vi "Data_get.vi"() -> ()   [LabVIEW 2009]
uses:
  <vilib>/Analysis/2dsp.llb/Real FFT.vi
  <vilib>/Analysis/NI_AALPro.lvlib
panel:
  in  "FFT every#":u32=1 min=1 max=1000 step=1
  in  "#steps":u32
  in  "f step (MHz)":dbl=0.0003 min=0.00025 max=67.0 step=1e-06 format="%#.12f"
  in  "ps/point":T1(ring)
  in  "ns/div":T2(ring)
  out "Current sweep":u32=1 min=1 max=1000 step=1
  in  "Ext":string="ccd"
  out "f cur. (MHz)":string
  in  "Name":string="trace"
  in  "Folder":path
  in  "#Sweeps":u32=1 min=1 max=1000 step=1
  in  "Ampl. (dBm)":dbl min=-135.0 max=30.0 step=0.5 format="%#_8g"
  in  "f start (MHz)":dbl=0.0003 min=0.00025 max=67.0 step=1e-06 format="%#.12f"
  in  "Start":bool
  in  "Quit":bool
  in  "E8257D VISA Port":refnum<visa-resource-name>="GPIB0::1::INSTR"
  out "read time (ms)":u32
  out "#points":u32
  out "Busy":bool
  in  "Repetition rate (Hz)":ext=2.5
  in  "Chirp start (MHz)":ext=2.5
  in  "Filter up to (MHz)":ext=2.5
  in  "Amount of averagings":u32=10
  out "Data":dbl[](array[numeric])
  out "XY Graph 5":cluster{ext[], dbl[]}(graph)
  out "FFT (Im)":dbl[](array[numeric])
  out "FFT (Re)":dbl[](array[numeric])
  out "Final array":ext[][](array[numeric])
  out "size(s)":i32
  out "Oscilloscope Data":dbl[](array[numeric])
  in  "Channel Number":u16=1
  out "Oscilloscope graph":dbl[](graph)
  in  "Stop":bool
  in  "TDS VISA Port":refnum<visa-resource-name>="GPIB0::1::INSTR"
  # "TDS6000"
  # "E8257D"
  # "File Storage"
  # "Control"
  # "Spectrum data"
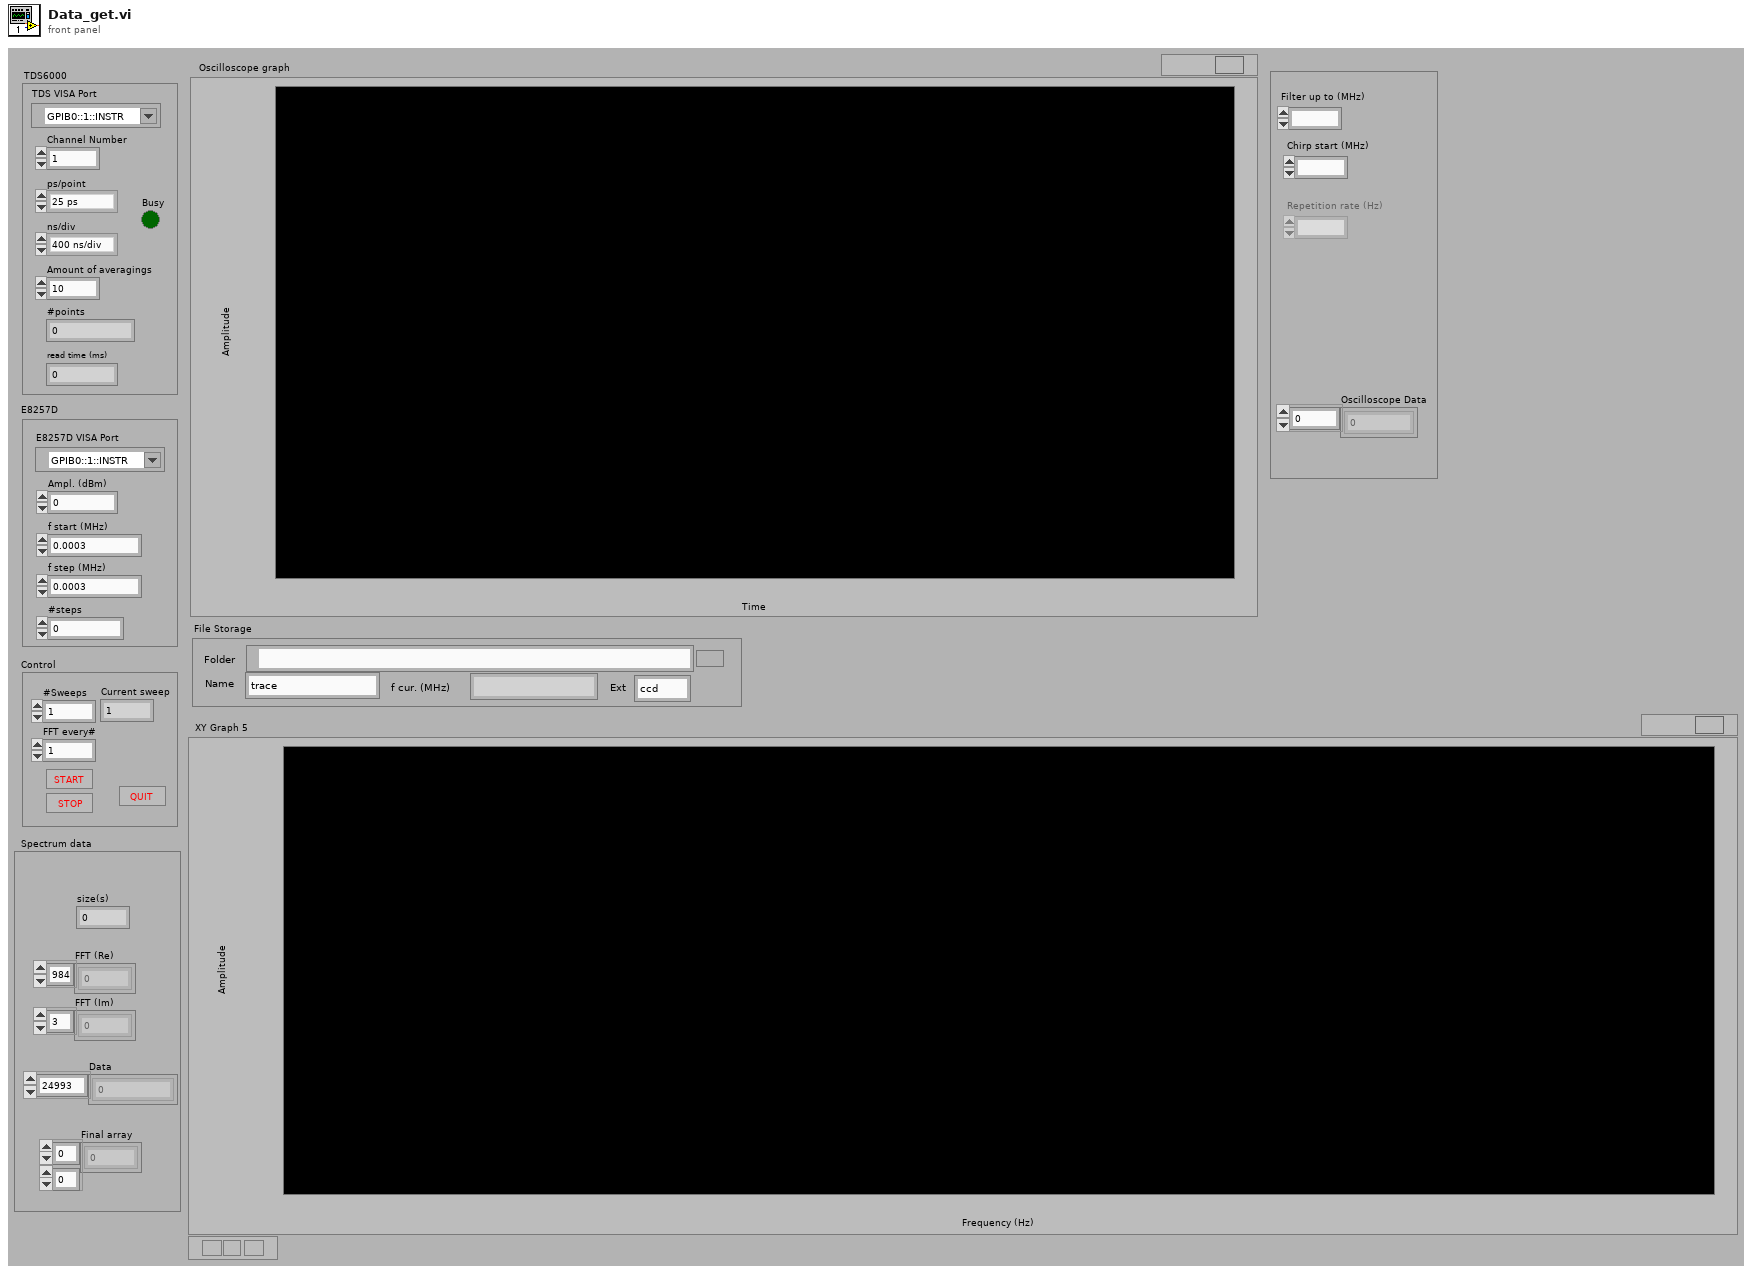
[diagram p1: front panel]
types:
  T1 = enum16{"25 ps", "50 ps", "100 ps", "200 ps", "400 ps", "800 ps", "2 ns"}
  T2 = enum16{"400 ns/div", "1 us/div", "2 us/div", "4 us/div", "10 us/div", "20 us/div"}
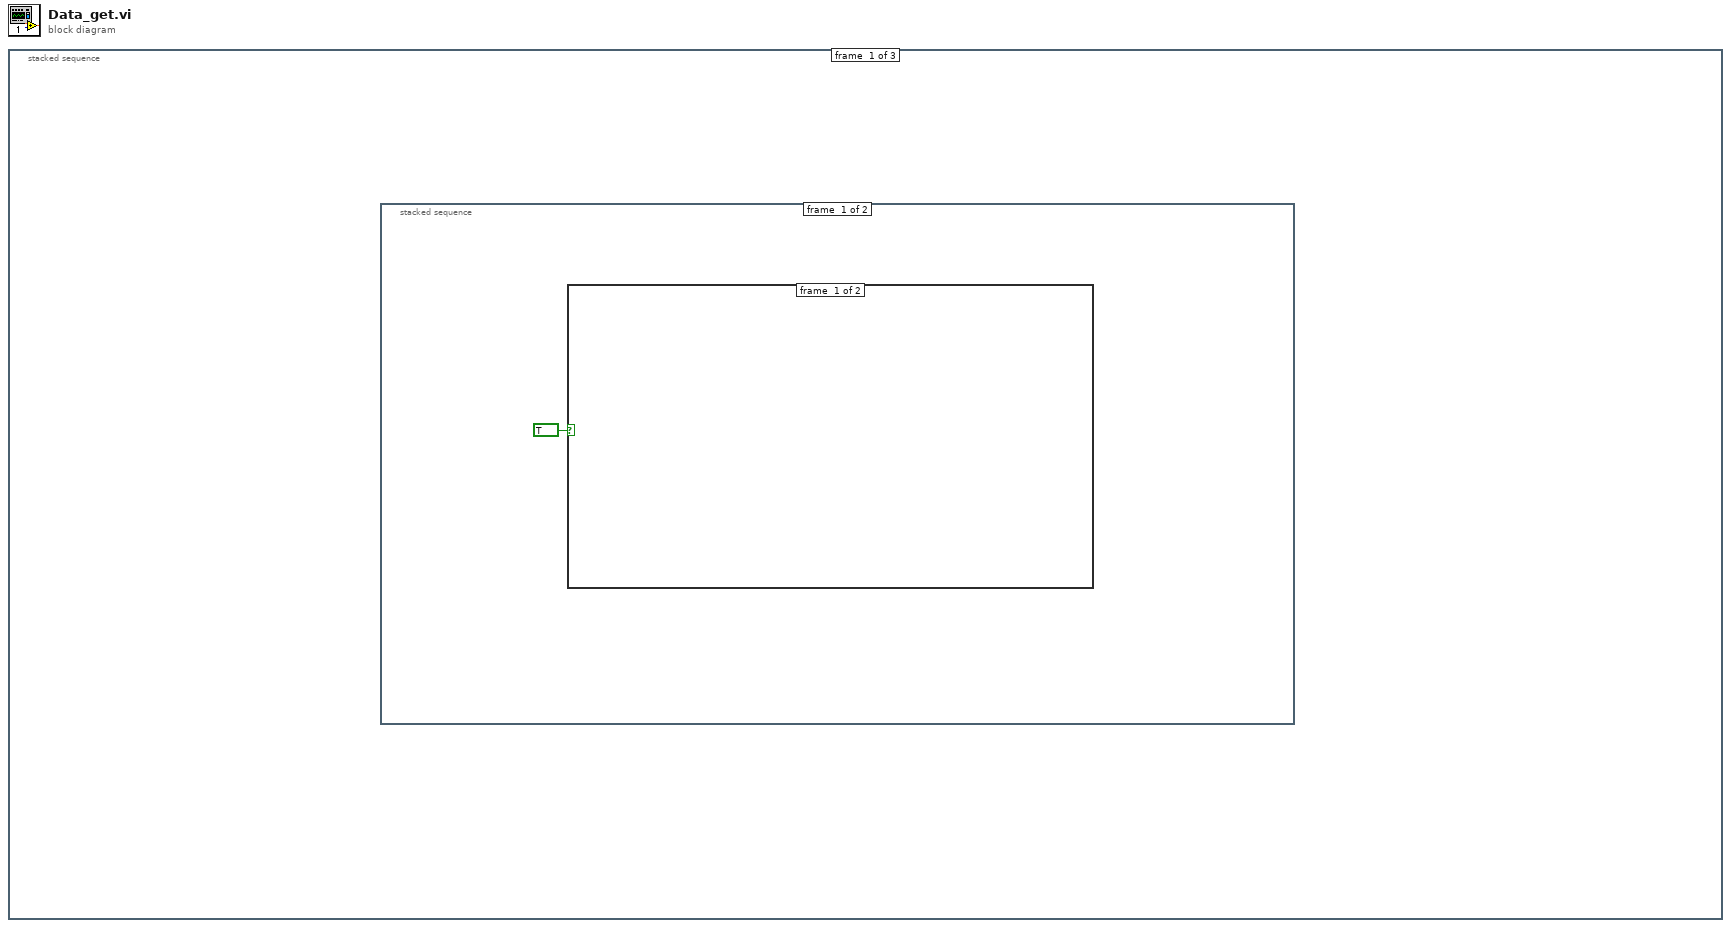
[diagram p0: block diagram]
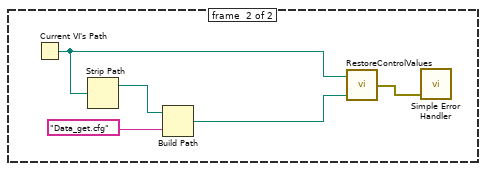
[diagram p2: hidden frame]
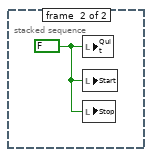
[diagram p3: hidden frame]
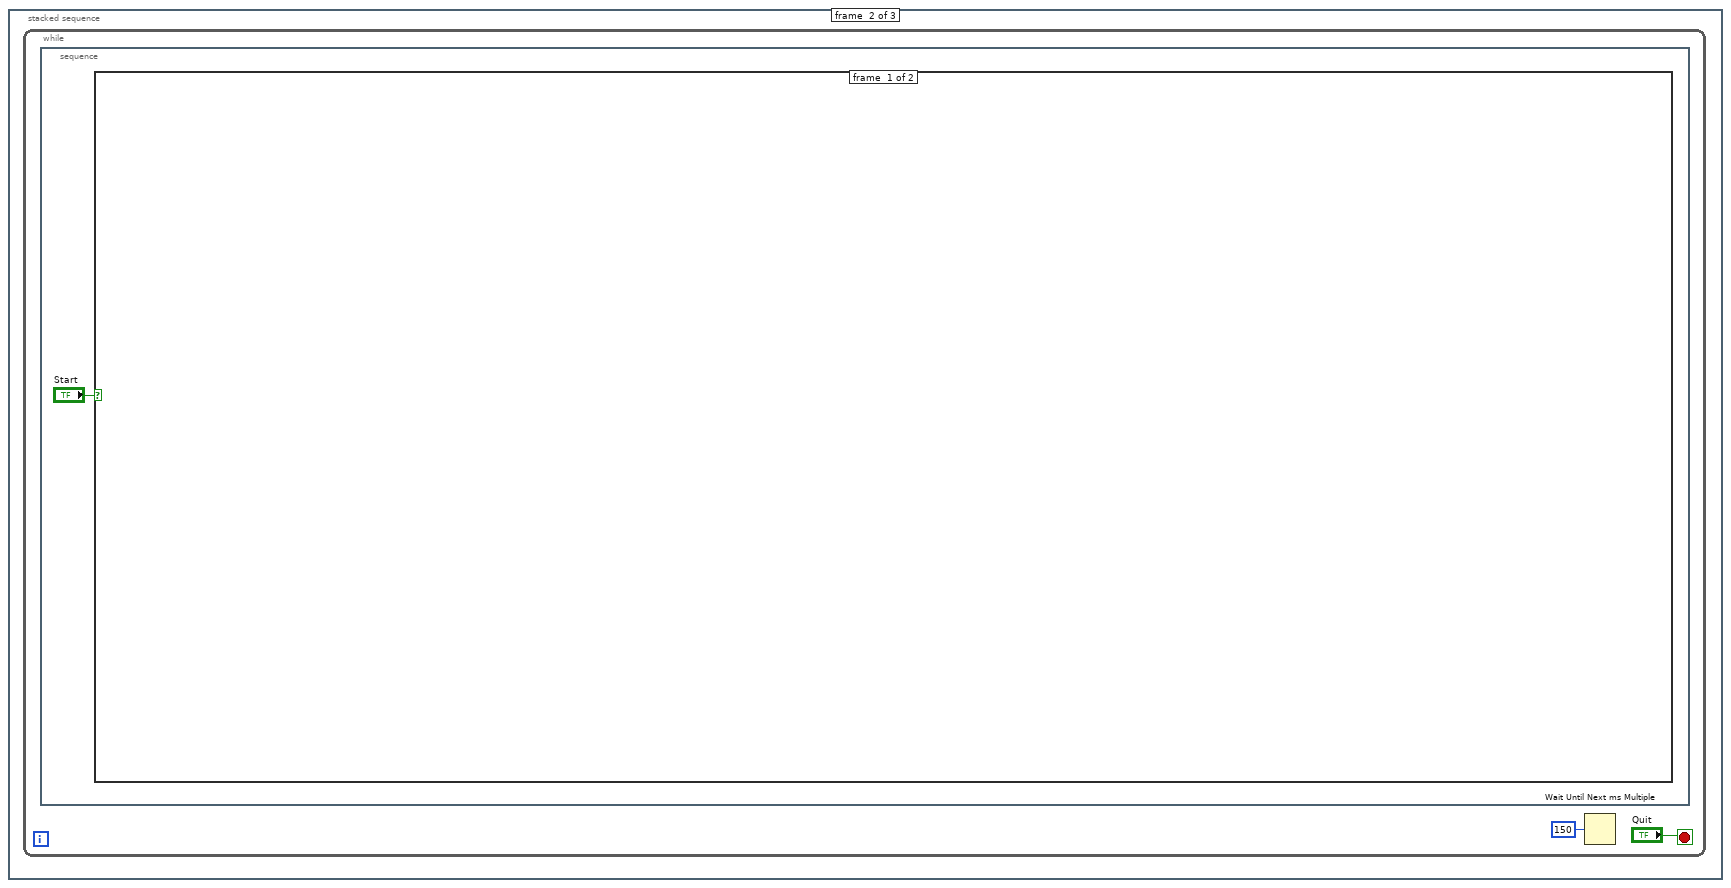
[diagram p4: hidden frame]
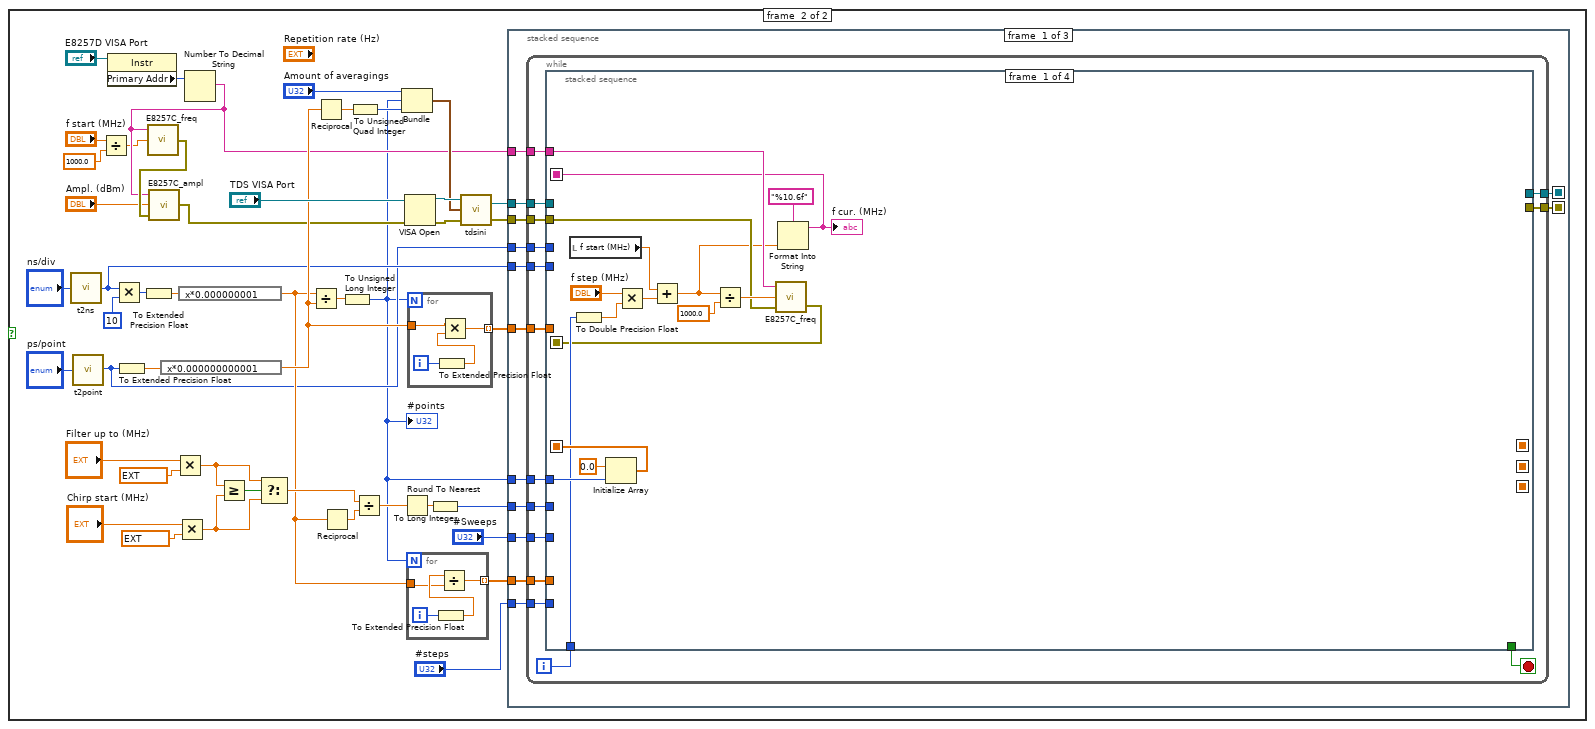
[diagram p5: hidden frame]
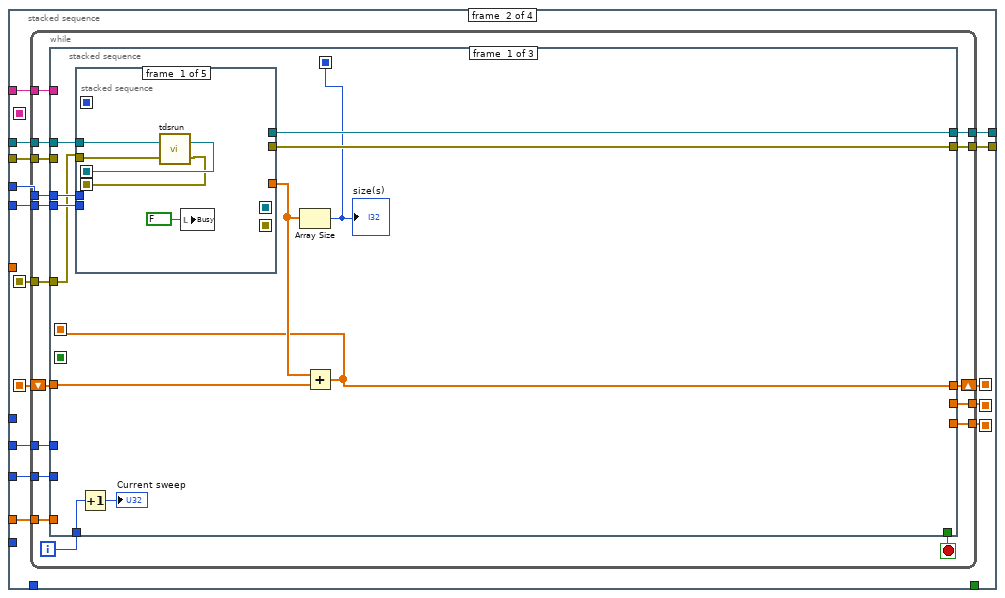
[diagram p6: hidden frame]
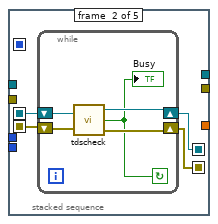
[diagram p7: hidden frame]
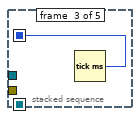
[diagram p8: hidden frame]
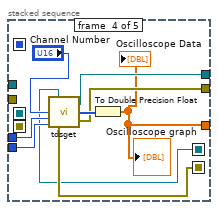
[diagram p9: hidden frame]
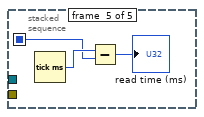
[diagram p10: hidden frame]
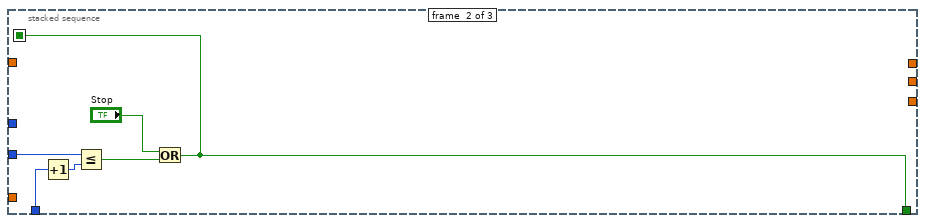
[diagram p11: hidden frame]
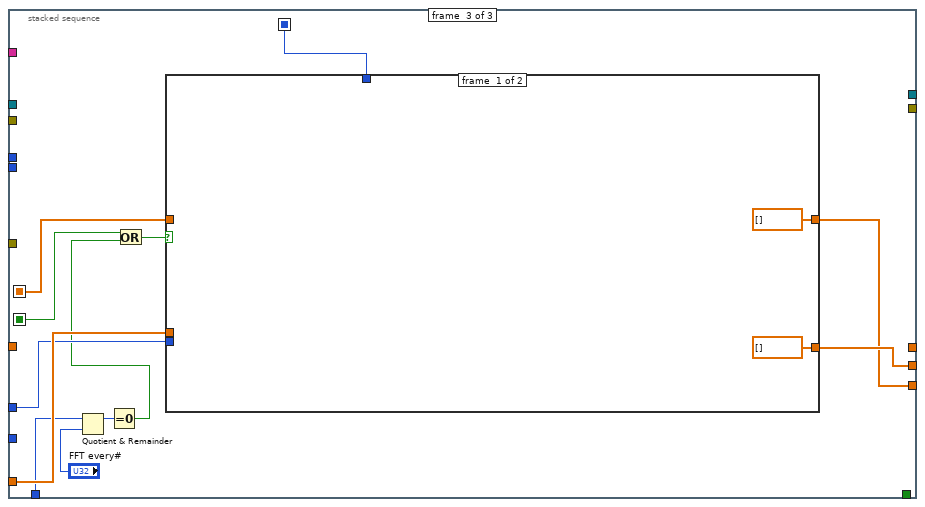
[diagram p12: hidden frame]
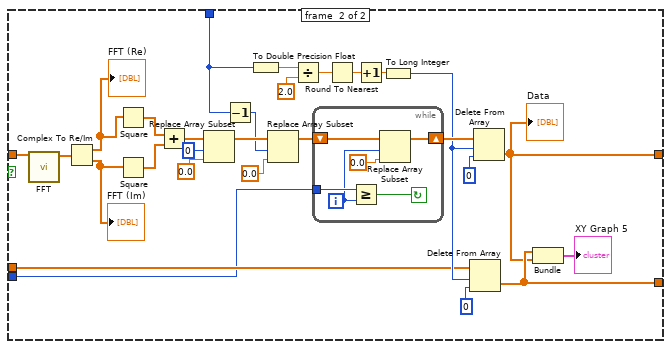
[diagram p13: hidden frame]
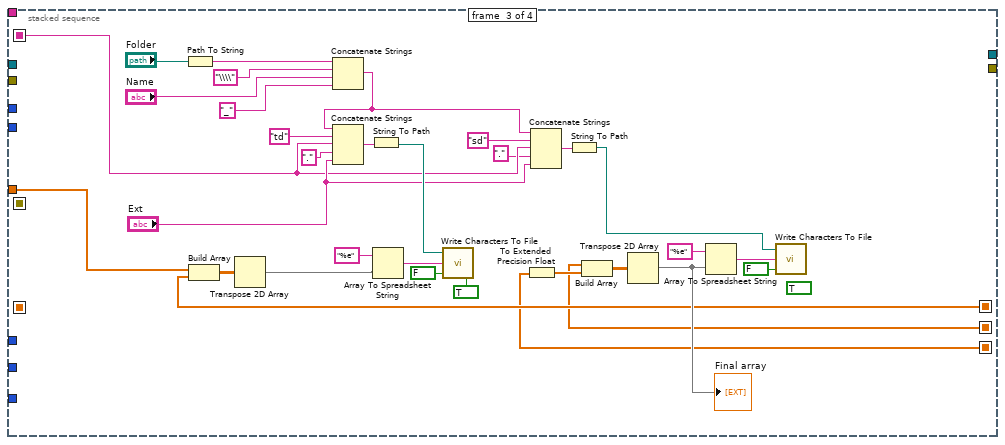
[diagram p14: hidden frame]
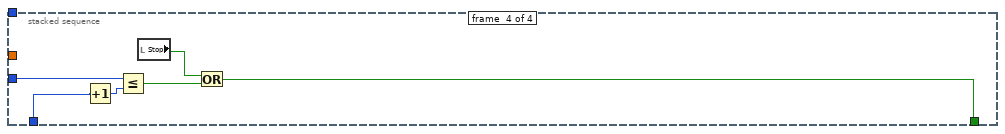
[diagram p15: hidden frame]
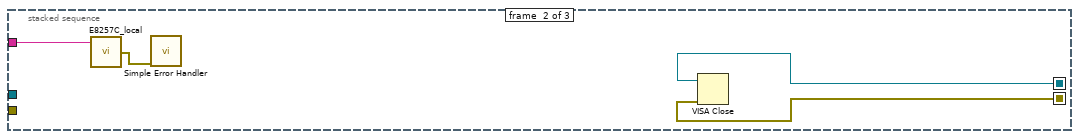
[diagram p16: hidden frame]
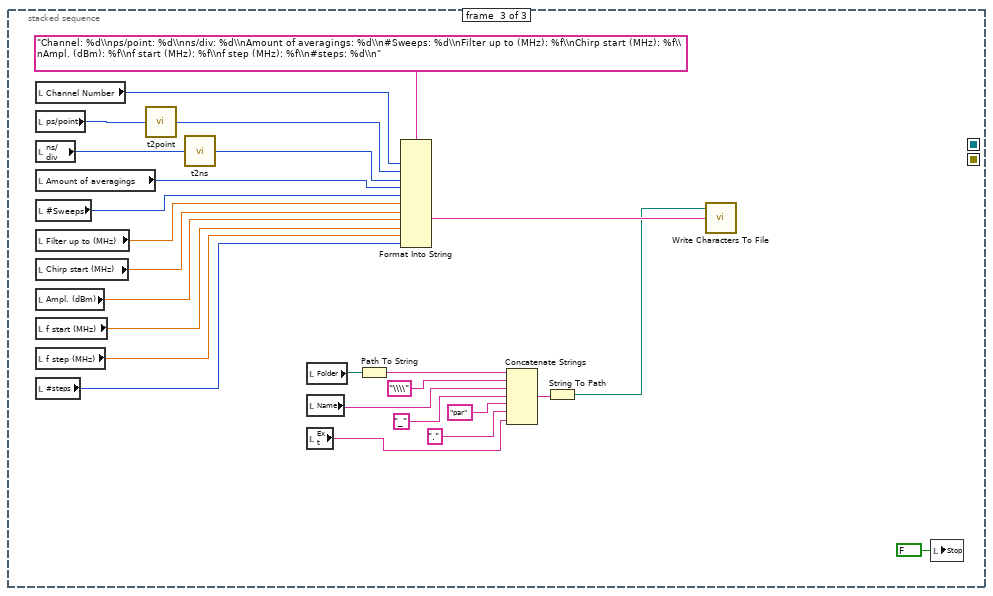
[diagram p17: hidden frame]
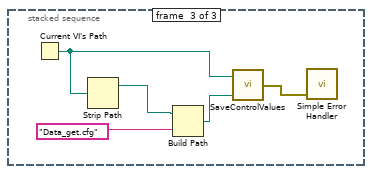
[diagram p18: hidden frame]
diagram:
  n1 = stacked-sequence {
    frame #0 {
      n2 = stacked-sequence {
        frame #0 {
          n3 = case shown="True" TRUE {
            frame #0 {
            }
            frame #1 {
              n4 = Current VI's Path() -> (path=w2:path)
              n5 = Strip Path(path=w2) -> (stripped path=w3:path)  [unwired: 1 out]
              n6 = Build Path(base path=w3, name or relative path="Data_get.cfg") -> (appended path=w5:path)
              n7 = call "RestoreControlValues.vi"("file path"=w5, "vi path"=w2) -> ("error out"=w4:errorcluster)
              n8 = call <vilib>:"Simple Error Handler.vi"("error in (no error)"=w4) -> ()  [unwired: 4 in, 5 out]
            }
          }
        }
        frame #1 {
          w7 = FALSE ("Quit")
          n9 = local write "Quit"(w7) -> ()
          n10 = local write "Start"(w7) -> ()
          n11 = local write "Stop"(w7) -> ()
        }
      }
    }
    frame #1 {
      n12 = while {
        stop <- "Quit" stop-if-true
        n13 = stacked-sequence {
          frame #0 {
            n14 = case shown="True" "Start" {
              frame #0 {
              }
              frame #1 {
                n15 = call "t2ns.vi"("t/div"="ns/div") -> ("ns/div"=w16:u32)
                n16 = call "t2point.vi"("t/point"="ps/point") -> ("ps/point"=w14:u32)
                n17 = Divide(x="f start (MHz)", y=1000.0) -> (x/y=w19:dbl)
                n18 = property class="Instr"(reference="E8257D VISA Port") -> ("Primary Addr"=w26:u16)  [unwired: 1 in, 2 out]
                n19 = Multiply(x=w16, y=u32 10) -> (x*y=w50:u32)
                n20 = To Extended Precision Float(1:w14) -> (0:w47:ext)
                n21 = To Extended Precision Float(1:w50) -> (0:w48:ext)
                n22 = expression code="x*0.000000000001"(w47) -> (w32:ext)
                n23 = Multiply(x="Filter up to (MHz)", y=ext 1000000.0) -> (x*y=w38:ext)
                n24 = Multiply(x="Chirp start (MHz)", y=ext 1000000.0) -> (x*y=w35:ext)
                n25 = expression code="x*0.000000001"(w48) -> (w28:ext)
                n26 = Number To Decimal String(number=w26) -> (decimal integer string=w23:string)  [unwired: 1 in]
                n27 = call "E8257C_freq.vi"("Frequency GHz"=w19, "GPIB address"=w23) -> ("error out"=w24:errorcluster)  [unwired: 1 in]
                n28 = call "E8257C_ampl.vi"("error in"=w24, "Amplitude dBm"="Ampl. (dBm)", "GPIB address"=w23) -> ("error out"=w22:errorcluster)
                n29 = Greater Or Equal?(x=w38, y=w35) -> (x >= y?=w46:bool)
                n30 = Select(t=w38, s=w46, f=w35) -> (s? t:f=w44:ext)
                n31 = Divide(x=w28, y=w32) -> (x/y=w49:ext)
                n32 = Reciprocal(x=w32) -> (1/x=w30:ext)
                n33 = Reciprocal(x=w28) -> (1/x=w45:ext)
                n34 = To Unsigned Long Integer(number=w49) -> (unsigned 32bit integer=w12:u32)
                "#points" <- w12
                n35 = To Unsigned Quad Integer(1:w30) -> (0:w31:u64)
                n36 = Divide(x=w44, y=w45) -> (x/y=w43:ext)
                n37 = Bundle("Amount of averagings"="Amount of averagings", w12, w31) -> (w33:cluster{"Amount of averagings ":u32, u32, u64})  [unwired: 1 in]
                n38 = Round To Nearest(number=w43) -> (nearest integer value=w42:ext)
                n39 = VISA Open(error in (no error)=w22, VISA resource name="TDS VISA Port") -> (VISA resource name=w53:refnum<visa-resource-name>, error out=w54:errorcluster)  [unwired: 3 in]
                n40 = for {
                  N: w12 -> [_]
                  tunnel: w28 -> [w294]
                  tunnel: [w296] -> w29 mode=indexing
                  i -> [w297]
                  n41 = To Extended Precision Float(1:w297) -> (0:w295:ext)
                  n42 = Divide(x=w295, y=w294) -> (x/y=w296:ext)
                }
                n43 = for {
                  N: w12 -> [_]
                  tunnel: w32 -> [w299]
                  tunnel: [w298] -> w17 mode=indexing
                  i -> [w301]
                  n44 = To Extended Precision Float(1:w301) -> (0:w300:ext)
                  n45 = Multiply(x=w299, y=w300) -> (x*y=w298:ext)
                }
                n46 = To Long Integer(number=w42) -> (32bit integer=w41:i32)
                n47 = call "tdsini.vi"("Error In (No Error)"=w54, "Acq_par"=w33, "VISA Port In"=w53) -> ("Error Out"=w55:errorcluster, "VISA Port Out"=w56:refnum<visa-resource-name>)
                n48 = stacked-sequence {
                  seq-local: [w61 _ _] -> [_ w267 _]
                  seq-local: [w60 _ _] -> [_ w266 _]
                  tunnel: w56 -> [w69 _ _]
                  tunnel: w55 -> [w68 _ _]
                  tunnel: w14 -> [w67 _ _]
                  tunnel: w16 -> [w66 _ _]
                  tunnel: w41 -> [w65 _ _]
                  tunnel: w29 -> [w64 _ _]
                  tunnel: w23 -> [w63 w264 _]
                  tunnel: "#Sweeps" -> [w62 _ _]
                  tunnel: w17 -> [w57 _ _]
                  tunnel: w12 -> [w59 _ _]
                  tunnel: "#steps" -> [w58 _ _]
                  frame #0 {
                    n49 = while {
                      tunnel: w69 -> [w84]
                      tunnel: w68 -> [w83]
                      tunnel: w67 -> [w82]
                      tunnel: w66 -> [w81]
                      tunnel: w65 -> [w80]
                      tunnel: w64 -> [w79]
                      tunnel: w63 -> [w78]
                      tunnel: w62 -> [w77]
                      tunnel: [w76] -> w61
                      tunnel: [w75] -> w60
                      tunnel: w59 -> [w74]
                      tunnel: w58 -> [w72]
                      tunnel: w57 -> [w70]
                      i -> [w73]
                      stop <- w71 stop-if-true
                      n50 = stacked-sequence {
                        seq-local: [w99 _ _ _] -> [_ w105 _ _]
                        seq-local: [w88 _ _ _] -> [_ w104 _ _]
                        seq-local: [_ w103 _ _] -> [_ _ w232 _]
                        seq-local: [_ w102 _ _] -> [_ _ w231 _]
                        seq-local: [_ w101 _ _] -> [_ _ w230 _]
                        seq-local: [w85 _ _ _] -> [_ _ w227 _]
                        tunnel: w84 -> [_ w115 _ _]
                        tunnel: w83 -> [w89 w114 _ _]
                        tunnel: w82 -> [_ w113 _ _]
                        tunnel: w81 -> [_ w112 _ _]
                        tunnel: w80 -> [_ w111 _ _]
                        tunnel: w79 -> [_ w110 _ _]
                        tunnel: w78 -> [w90 w109 _ _]
                        tunnel: w77 -> [_ w108 _ _]
                        tunnel: [_ w107 _ _] -> w76
                        tunnel: [_ w106 _ _] -> w75
                        tunnel: w74 -> [w98 _ _ _]
                        tunnel: w73 -> [w93 _ _ w260]
                        tunnel: w72 -> [_ _ _ w259]
                        tunnel: [_ _ _ w258] -> w71
                        tunnel: w70 -> [_ _ w233 _]
                        frame #0 {
                          n51 = local read "f start (MHz)"() -> (w91:dbl)
                          n52 = To Double Precision Float(number=w93) -> (double precision float=w94:dbl)
                          n53 = Initialize Array(0.0 ("element"), w98) -> (w99:dbl[])
                          n54 = Multiply(x="f step (MHz)", y=w94) -> (x*y=w92:dbl)
                          n55 = Add(x=w91, y=w92) -> (x+y=w87:dbl)
                          n56 = Divide(x=w87, y=1000.0) -> (x/y=w97:dbl)
                          n57 = call "E8257C_freq.vi"("error in"=w89, "Frequency GHz"=w97, "GPIB address"=w90) -> ("error out"=w88:errorcluster)
                          n58 = Format Into String(format string="%10.6f", w87) -> (resulting string=w85:string)  [unwired: 2 in, 1 out]
                          "f cur. (MHz)" <- w85
                        }
                        frame #1 {
                          n59 = while {
                            tunnel: [w129] -> w106
                            tunnel: [w130] -> w107
                            tunnel: w114 -> [w131]
                            tunnel: w115 -> [w132]
                            tunnel: w113 -> [w128]
                            tunnel: w112 -> [w127]
                            tunnel: w110 -> [w125]
                            tunnel: w111 -> [w126]
                            tunnel: w109 -> [w122]
                            tunnel: w108 -> [w121]
                            shift-right: [w119] -> w103
                            shift-left: w105 -> [w120]
                            tunnel: [w118] -> w102
                            tunnel: w104 -> [w117]
                            tunnel: [w116] -> w101
                            i -> [w124]
                            stop <- w123 stop-if-true
                            n60 = stacked-sequence {
                              seq-local: [w133 _ _] -> [_ _ w189]
                              seq-local: [w134 _ _] -> [_ _ w188]
                              seq-local: [_ w172 _] -> [_ _ w179]
                              tunnel: w132 -> [w144 _ _]
                              tunnel: w131 -> [_ _ _]
                              tunnel: [w143 _ _] -> w130
                              tunnel: [w142 _ _] -> w129
                              tunnel: w128 -> [w141 _ _]
                              tunnel: w127 -> [w140 _ _]
                              tunnel: w126 -> [_ _ w186]
                              tunnel: w125 -> [_ _ w187]
                              tunnel: w124 -> [w137 w177 w183]
                              tunnel: [_ w172 _] -> w123
                              tunnel: w122 -> [_ _ _]
                              tunnel: w121 -> [_ w174 _]
                              tunnel: w120 -> [w139 _ _]
                              tunnel: [w134 _ _] -> w119
                              tunnel: [_ _ w185] -> w118
                              tunnel: w117 -> [w136 _ _]
                              tunnel: [_ _ w184] -> w116
                              frame #0 {
                                n61 = stacked-sequence {
                                seq-local: [w147 _ _ _ _] -> [_ w153 _ _ _]
                                seq-local: [w146 _ _ _ _] -> [_ w152 _ _ _]
                                seq-local: [_ w150 _ _ _] -> [_ _ _ w161 _]
                                seq-local: [_ w151 _ _ _] -> [_ _ _ w160 _]
                                seq-local: [_ _ w159 _ _] -> [_ _ _ _ w170]
                                tunnel: w144 -> [w148 _ _ _ _]
                                tunnel: w136 -> [w149 _ _ _ _]
                                tunnel: [_ _ _ w167 _] -> w143
                                tunnel: [_ _ _ w166 _] -> w142
                                tunnel: w141 -> [_ _ _ w164 _]
                                tunnel: w140 -> [_ _ _ w163 _]
                                tunnel: [_ _ _ w162 _] -> w135
                                frame #0 {
                                n62 = call "tdsrun.vi"("Error In (No Error)"=w149, "VISA Port In"=w148) -> ("Error Out"=w146:errorcluster, "VISA Port Out"=w147:refnum<visa-resource-name>)
                                n63 = local write "Busy"(FALSE ("Busy")) -> ()
                                }
                                frame #1 {
                                n64 = while {
                                shift-right: [w156] -> w151
                                shift-left: w153 -> [w157]
                                shift-right: [w155] -> w150
                                shift-left: w152 -> [w158]
                                stop <- w154 continue-if-true
                                n65 = call "tdscheck.vi"("VISA Port In"=w157, "Error In (No Error)"=w158) -> ("VISA Port Out"=w156:refnum<visa-resource-name>, "busy"=w154:bool, "Error Out"=w155:errorcluster)
                                "Busy" <- w154
                                }
                                }
                                frame #2 {
                                n66 = Tick Count (ms)() -> (millisecond timer value=w159:u32)
                                }
                                frame #3 {
                                n67 = call "tdsget.vi"("VISA Port In"=w160, "Channel Number"="Channel Number", "ps/point"=w164, "ns/div"=w163, "Error In (No Error)"=w161) -> ("VISA Port Out"=w167:refnum<visa-resource-name>, "TDS Data"=w168:u16[], "Error Out"=w166:errorcluster)  [unwired: 8 in]
                                n68 = To Double Precision Float(number=w168) -> (double precision float=w162:dbl[])
                                "Oscilloscope graph" <- w162
                                "Oscilloscope Data" <- w162
                                }
                                frame #4 {
                                n69 = Tick Count (ms)() -> (millisecond timer value=w171:u32)
                                n70 = Subtract(x=w171, y=w170) -> (x-y=→"read time (ms)":u32)
                                }
                                }
                                n71 = Increment(x=w137) -> (x+1=→"Current sweep":i32)
                                n72 = Array Size(array=w135) -> (size(s)=w133:i32)
                                "size(s)" <- w133
                                n73 = Add(x=w135, y=w139) -> (x+y=w134:dbl[])
                              }
                              frame #1 {
                                n74 = Increment(x=w177) -> (x+1=w173:i32)
                                n75 = Less Or Equal?(x=w174, y=w173) -> (x <= y?=w176:bool)
                                n76 = Or(x="Stop", y=w176) -> (x .or. y?=w172:bool)
                              }
                              frame #2 {
                                n77 = Quotient & Remainder(x=w183, y="FFT every#") -> (x-y*floor(x/y)=w181:u32)  [unwired: 1 out]
                                n78 = Equal To 0?(x=w181) -> (x = 0?=w178:bool)
                                n79 = Or(x=w179, y=w178) -> (x .or. y?=w180:bool)
                                n80 = case shown="True" w180 {
                                tunnel: w189 -> [_ w197]
                                tunnel: w188 -> [_ w196]
                                tunnel: w187 -> [_ w195]
                                tunnel: w186 -> [_ w194]
                                tunnel: [ext[] [] w193] -> w185
                                tunnel: [dbl[] [] w192] -> w184
                                frame #0 {
                                }
                                frame #1 {
                                n81 = call-poly <vilib>:"FFT.vi"("X"=w196) -> ("FFT {X}"=w219:cdb[])  [unwired: 9 in, 1 out]
                                n82 = Complex To Re/Im(x + iy=w219) -> (x=w218:dbl[], y=w217:dbl[])
                                "FFT (Re)" <- w218
                                "FFT (Im)" <- w217
                                n83 = Square(x=w218) -> (x^2=w216:dbl[])
                                n84 = Square(x=w217) -> (x^2=w215:dbl[])
                                n85 = Add(x=w216, y=w215) -> (x+y=w211:dbl[])
                                n86 = Replace Array Subset(array=w211, new element=0.0 ("new element/subarray"), index=0) -> (w210:dbl[])
                                n87 = Decrement(x=w197) -> (x-1=w209:i32)
                                n88 = To Double Precision Float(number=w197) -> (double precision float=w205:dbl)
                                n89 = Replace Array Subset(array=w210, new element=0.0 ("new element/subarray"), index=w209) -> (w207:dbl[])
                                n90 = Divide(x=w205, y=2.0) -> (x/y=w203:dbl)
                                n91 = while {
                                tunnel: w194 -> [w224]
                                shift-right: [w222] -> w206
                                shift-left: w207 -> [w223]
                                i -> [w221]
                                stop <- w225 continue-if-true
                                n92 = Greater Or Equal?(x=w224, y=w221) -> (x >= y?=w225:bool)
                                n93 = Replace Array Subset(array=w223, new element=0.0 ("new element/subarray"), index=w221) -> (w222:dbl[])
                                }
                                n94 = Round To Nearest(number=w203) -> (nearest integer value=w202:dbl)
                                n95 = Increment(x=w202) -> (x+1=w201:dbl)
                                n96 = To Long Integer(number=w201) -> (32bit integer=w198:i32)
                                n97 = Delete From Array(array=w195, length=w198, index=0) -> (deleted portion=w193:ext[])  [unwired: 1 out]
                                n98 = Delete From Array(array=w206, length=w198, index=0) -> (deleted portion=w192:dbl[])  [unwired: 1 out]
                                "Data" <- w192
                                n99 = Bundle(w193, w192) -> (→"XY Graph 5":cluster{ext[], dbl[]})  [unwired: 1 in]
                                }
                                }
                              }
                            }
                          }
                        }
                        frame #2 {
                          (unwired) TRUE
                          n100 = Path To String(path="Folder") -> (string=w251:string)
                          n101 = Build Array(w233, w232) -> (w252:ext[][])
                          n102 = Transpose 2D Array(2D array=w252) -> (transposed array=w239:ext[][])
                          n103 = Concatenate Strings(w251, "\\\\" ("string"), "Name", "_") -> (w235:string)
                          n104 = Concatenate Strings(w235, "td", w227, ".", "Ext") -> (w245:string)
                          n105 = String To Path(string=w245) -> (path=w240:path)
                          n106 = Array To Spreadsheet String(array=w239, 3:"%e") -> (spreadsheet string=w242:string)  [unwired: 1 in]
                          n107 = call <vilib>:"Write Characters To File.vi"("convert eol? (no:F)"=TRUE, "append to file? (new file:F)"=FALSE, "character string"=w242, "file path (dialog if empty)"=w240) -> ()  [unwired: 1 in, 1 out]
                          n108 = To Extended Precision Float(1:w230) -> (0:w253:ext[])
                          n109 = Concatenate Strings(w235, "sd", w227, ".", "Ext") -> (w237:string)
                          n110 = String To Path(string=w237) -> (path=w236:path)
                          n111 = Build Array(w231, w253) -> (w229:ext[][])
                          n112 = Transpose 2D Array(2D array=w229) -> (transposed array=w256:ext[][])
                          "Final array" <- w256
                          n113 = Array To Spreadsheet String(array=w256, 3:"%e") -> (spreadsheet string=w254:string)  [unwired: 1 in]
                          n114 = call <vilib>:"Write Characters To File.vi"("append to file? (new file:F)"=FALSE, "character string"=w254, "file path (dialog if empty)"=w236) -> ()  [unwired: 2 in, 1 out]
                        }
                        frame #3 {
                          n115 = Increment(x=w260) -> (x+1=w262:i32)
                          n116 = Less Or Equal?(x=w259, y=w262) -> (x <= y?=w263:bool)
                          n117 = local read "Stop"() -> (w261:bool)
                          n118 = Or(x=w261, y=w263) -> (x .or. y?=w258:bool)
                        }
                      }
                    }
                  }
                  frame #1 {
                    n119 = call "E8257C_local.vi"("GPIB address"=w264) -> ("error out"=w265:errorcluster)  [unwired: 1 in]
                    n120 = call <vilib>:"Simple Error Handler.vi"("error in (no error)"=w265) -> ()  [unwired: 4 in, 5 out]
                    n121 = VISA Close(VISA resource name=w267, error in (no error)=w266) -> ()  [unwired: 1 out]
                  }
                  frame #2 {
                    n122 = local read "Channel Number"() -> (w291:u16)
                    n123 = local read "ps/point"() -> (w290:T1)
                    n124 = local read "ns/div"() -> (w289:T2)
                    n125 = local read "Amount of averagings"() -> (w288:u32)
                    n126 = local read "#Sweeps"() -> (w286:u32)
                    n127 = local read "Filter up to (MHz)"() -> (w285:ext)
                    n128 = local read "Chirp start (MHz)"() -> (w284:ext)
                    n129 = local read "Ampl. (dBm)"() -> (w283:dbl)
                    n130 = local read "f start (MHz)"() -> (w280:dbl)
                    n131 = local read "f step (MHz)"() -> (w279:dbl)
                    n132 = local read "#steps"() -> (w278:u32)
                    n133 = call "t2point.vi"("t/point"=w290) -> ("ps/point"=w281:u32)
                    n134 = call "t2ns.vi"("t/div"=w289) -> ("ns/div"=w282:u32)
                    n135 = local read "Folder"() -> (w274:path)
                    n136 = local read "Name"() -> (w273:string)
                    n137 = local read "Ext"() -> (w270:string)
                    n138 = Path To String(path=w274) -> (string=w277:string)
                    n139 = Format Into String(format string="Channel: %d\\nps/point: %d\\nns/div: %d\\nAmount of averagings: %d\\n#Sweeps: %d\\nFilter up to (MHz): %f\\nChirp start (MHz): %f\\nAmpl. (dBm): %f\\nf start (MHz): %f\\nf step (MHz): %f\\n#steps: %d\\n", w291, w281, w282, w288, w286, w285, w284, w283, w280, w279, w278) -> (resulting string=w293:string)  [unwired: 2 in, 1 out]
                    n140 = Concatenate Strings(w277, "\\\\" ("string"), w273, "_", "par", ".", w270) -> (w269:string)
                    n141 = String To Path(string=w269) -> (path=w268:path)
                    n142 = call <vilib>:"Write Characters To File.vi"("character string"=w293, "file path (dialog if empty)"=w268) -> ()  [unwired: 3 in, 1 out]
                    n143 = local write "Stop"(FALSE ("Stop")) -> ()
                  }
                }
              }
            }
          }
        }
        n144 = Wait Until Next ms Multiple(millisecond multiple=u32 150) -> ()  [unwired: 1 out]
      }
    }
    frame #2 {
      n145 = Current VI's Path() -> (path=w302:path)
      n146 = Strip Path(path=w302) -> (stripped path=w303:path)  [unwired: 1 out]
      n147 = Build Path(base path=w303, name or relative path="Data_get.cfg") -> (appended path=w305:path)
      n148 = call "SaveControlValues.vi"("file path"=w305, "vi path"=w302) -> ("error out"=w304:errorcluster)
      n149 = call <vilib>:"Simple Error Handler.vi"("error in (no error)"=w304) -> ()  [unwired: 4 in, 5 out]
    }
  }
